vi "Configure DC Input Impedance.vi"(8 "error in (no error)":errorcluster, 10 "DC Input Impedance (0 : 10M)":i32(ring) items=["10M", "10G"], 11 "VISA resource name":refnum<visa-resource-name>) -> (0 "error out":errorcluster, 3 "VISA resource name out":refnum<visa-resource-name>)   [LabVIEW 2021, in "GWInstek  GDM8351.lvlib"]
doc: "Sets the input impedance for DC voltage.\n\n<B>Note</B>\nonly 100mV and 1V range."
uses:
  <instrlib>/GWInstek  GDM8351/GWInstek  GDM8351.lvlib
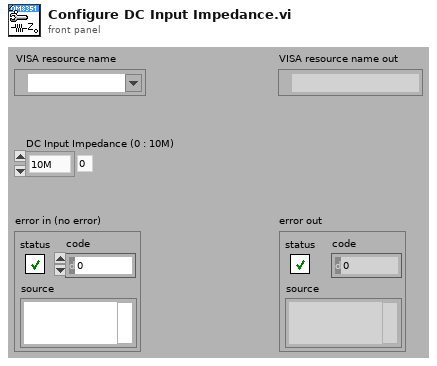
[diagram p1: front panel]
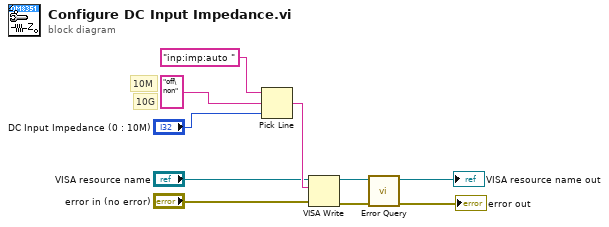
[diagram p0: block diagram]
diagram:
  # "10G"
  # "10M"
  n1 = Pick Line(string ("")="inp:imp:auto ", multi-line string="off\non", line index="DC Input Impedance (0 : 10M)") -> (output string=w7:string)
  n2 = VISA Write(VISA resource name="VISA resource name", write buffer=w7, error in (no error)="error in (no error)") -> (VISA resource name out=w4:refnum<visa-resource-name>, error out=w3:errorcluster)  [unwired: 1 out]
  n3 = call <instrlib>:"Error Query.vi"("error in (no error)"=w3, "VISA resource name"=w4) -> ("error out"=→"error out":errorcluster, "VISA resource name out"=→"VISA resource name out":refnum<visa-resource-name>)  [unwired: 6 in, 2 out]
